vi "2 Ball Double Hot B.vi"(1 "Run?":bool) -> (0 "Done?":bool)   [LabVIEW 2013]
uses:
  Globals/Homes.vi
  Globals/Useful Values.vi
panel:
  out "Time Elapsed":dbl
  out "Sum":dbl
  out "Ready for Vision?":bool
  out "Side":dbl
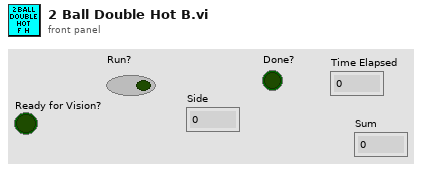
[diagram p1: front panel]
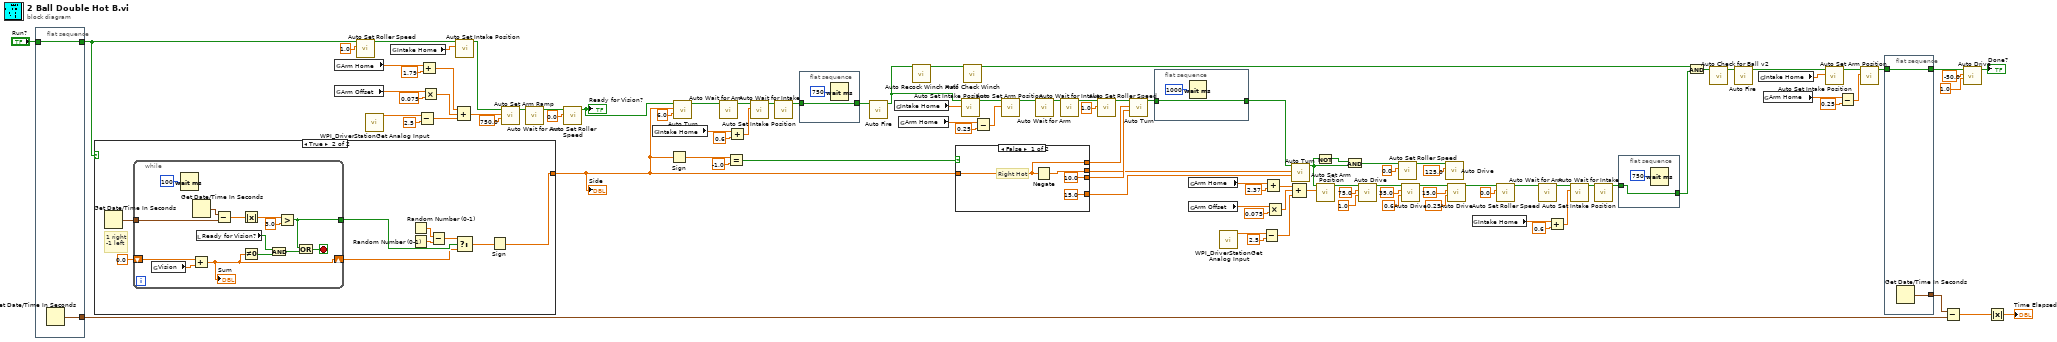
[diagram p0: block diagram]
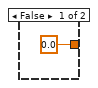
[diagram p2: hidden frame]
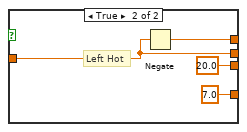
[diagram p3: hidden frame]
diagram:
  n1 = flat-sequence {
    tunnel: "Run?" -> [w107]
    tunnel: [w107] -> w49
    tunnel: [w106] -> w44
    frame #0 {
      n2 = Get Date/Time In Seconds() -> (seconds since 1Jan1904=w106:timestamp)
    }
  }
  n3 = case shown="True" w49 {
    tunnel: [0.0 w109] -> w54
    frame False {
    }
    frame True {
      # "1 right\n-1 left"
      n4 = Get Date/Time In Seconds() -> (seconds since 1Jan1904=w116:timestamp)
      n5 = while {
        shift-right: [w127] -> w111
        shift-left: 0.0 -> [w130]
        tunnel: w116 -> [w125]
        tunnel: [w118] -> w112
        stop <- w120 stop-if-true
        n6 = global read "Useful Values.vi" "Vision"() -> (w131:dbl)
        n7 = Wait (ms)(milliseconds to wait=u32 100) -> ()  [unwired: 1 out]
        n8 = Add(x=w130, y=w131) -> (x+y=w127:dbl)
        "Sum" <- w127
        n9 = Get Date/Time In Seconds() -> (seconds since 1Jan1904=w124:timestamp)
        n10 = local read "Ready for Vision?"() -> (w128:bool)
        n11 = Subtract(x=w124, y=w125) -> (x-y=w123:dbl)
        n12 = Absolute Value(x=w123) -> (abs(x)=w122:dbl)
        n13 = Not Equal To 0?(x=w127) -> (x != 0?=w126:bool)
        n14 = And(x=w128, y=w126) -> (x .and. y?=w119:bool)
        n15 = Greater?(x=w122, y=3.0) -> (0:w118:bool)
        n16 = Or(x=w118, y=w119) -> (x .or. y?=w120:bool)
      }
      n17 = Random Number (0-1)() -> (number: 0 to 1=w113:dbl)
      n18 = Random Number (0-1)() -> (number: 0 to 1=w114:dbl)
      n19 = Subtract(x=w113, y=w114) -> (x-y=w115:dbl)
      n20 = Select(t=w115, s=w112, f=w111) -> (s? t:f=w110:dbl)
      n21 = Sign(1:w110) -> (0:w109:dbl)
    }
  }
  "Side" <- w54
  n22 = global read "Homes.vi" "Arm Home"() -> (w9:dbl)
  n23 = global read "Useful Values.vi" "Arm Offset"() -> (w6:dbl)
  n24 = call "Auto Set Roller Speed.vi"("Value"=1.0, "Run?"=w49) -> ("Done"=w74:bool)  [unwired: 9 in]
  n25 = call <vilib>:"WPI_DriverStationGet Analog Input.vi"() -> ("Analog 1 (V)"=w3:dbl)  [unwired: 8 in, 3 out]
  n26 = global read "Homes.vi" "Intake Home"() -> (w104:dbl)
  n27 = Subtract(x=w3, y=2.5) -> (x-y=w2:dbl)
  n28 = Add(x=w9, y=1.79) -> (x+y=w5:dbl)
  n29 = Multiply(x=w6, y=0.075) -> (x*y=w8:dbl)
  n30 = call "Auto Set Intake Position.vi"("Intake Position"=w104, "Run?"=w74) -> ("Done"=w73:bool)  [unwired: 9 in]
  n31 = Compound Arithmetic op=ADD(w5, w8, w2) -> (w1:dbl)
  n32 = call "Auto Set Arm Ramp.vi"("Time (ms)"=750.0, "Arm Position"=w1, "Run?"=w73) -> ("Done"=w52:bool)  [unwired: 8 in]
  n33 = call "Auto Wait for Arm.vi"("Run?"=w52) -> ("Done"=w53:bool)  [unwired: 10 in]
  n34 = call "Auto Set Roller Speed.vi"("Value"=0.0, "Run?"=w53) -> ("Done"=w51:bool)  [unwired: 9 in]
  "Ready for Vision?" <- w51
  n35 = global read "Homes.vi" "Intake Home"() -> (w103:dbl)
  n36 = Sign(1:w54) -> (0:w91:dbl)
  n37 = call "Auto Turn.vi"("Turn Amount"=6.0, "+/-?"=w54, "Run?"=w51) -> ("Done"=w70:bool)  [unwired: 8 in]
  n38 = call "Auto Wait for Arm.vi"("Run?"=w70) -> ("Done"=w100:bool)  [unwired: 10 in]
  n39 = Equal?(x=w91, y=-1.0) -> (x = y?=w89:bool)
  n40 = Add(x=w103, y=0.6) -> (x+y=w102:dbl)
  n41 = call "Auto Set Intake Position.vi"("Intake Position"=w102, "Run?"=w100) -> ("Done"=w71:bool)  [unwired: 9 in]
  n42 = call "Auto Wait for Intake.vi"("Run?"=w71) -> ("Done"=w86:bool)  [unwired: 10 in]
  n43 = flat-sequence {
    tunnel: w86 -> [w132]
    tunnel: [w132] -> w77
    frame #0 {
      n44 = Wait (ms)(milliseconds to wait=u32 750) -> ()  [unwired: 1 out]
    }
  }
  n45 = call "Auto Fire.vi"("Run?"=w77) -> ("Done"=w68:bool)  [unwired: 10 in]
  n46 = global read "Homes.vi" "Intake Home"() -> (w98:dbl)
  n47 = global read "Homes.vi" "Arm Home"() -> (w81:dbl)
  n48 = call "Auto Recock Winch Half.vi"("Run?"=w68) -> ("Done"=w69:bool)  [unwired: 10 in]
  n49 = case shown="False" w89 {
    tunnel: [10.0 ("Turn Amount") 20.0 ("Turn Amount")] -> w88
    tunnel: w54 -> [w135 w138]
    tunnel: [w135 w139] -> w87
    tunnel: [w136 w138] -> w42
    tunnel: [15.0 ("Turn Amount") 7.0 ("Turn Amount")] -> w41
    frame False {
      # "Right Hot"
      n50 = Negate(x=w135) -> (-x=w136:dbl)
    }
    frame True {
      # "Left Hot"
      n51 = Negate(x=w138) -> (-x=w139:dbl)
    }
  }
  n52 = call "Auto Set Intake Position.vi"("Intake Position"=w98, "Run?"=w68) -> ("Done"=w99:bool)  [unwired: 9 in]
  n53 = call "Auto Check Winch.vi"("Run?"=w69) -> ("Done"=w33:bool)  [unwired: 10 in]
  n54 = Subtract(x=w81, y=0.25) -> (x-y=w80:dbl)
  n55 = call "Auto Set Arm Position.vi"("Arm Position"=w80, "Run?"=w99) -> ("Done"=w97:bool)  [unwired: 9 in]
  n56 = call "Auto Wait for Arm.vi"("Run?"=w97) -> ("Done"=w96:bool)  [unwired: 10 in]
  n57 = call "Auto Wait for Intake.vi"("Run?"=w96) -> ("Done"=w95:bool)  [unwired: 10 in]
  n58 = call "Auto Set Roller Speed.vi"("Value"=1.0, "Run?"=w95) -> ("Done"=w93:bool)  [unwired: 9 in]
  n59 = call "Auto Turn.vi"("Turn Amount"=w88, "+/-?"=w87, "Run?"=w93) -> ("Done"=w92:bool)  [unwired: 8 in]
  n60 = flat-sequence {
    tunnel: w92 -> [w143]
    tunnel: [w143] -> w43
    frame #0 {
      n61 = Wait (ms)(milliseconds to wait=u32 1000) -> ()  [unwired: 1 out]
    }
  }
  n62 = global read "Homes.vi" "Arm Home"() -> (w19:dbl)
  n63 = global read "Useful Values.vi" "Arm Offset"() -> (w16:dbl)
  n64 = call <vilib>:"WPI_DriverStationGet Analog Input.vi"() -> ("Analog 1 (V)"=w13:dbl)  [unwired: 8 in, 3 out]
  n65 = Subtract(x=w13, y=2.5) -> (x-y=w12:dbl)
  n66 = Add(x=w19, y=2.37) -> (x+y=w15:dbl)
  n67 = Multiply(x=w16, y=0.075) -> (x*y=w18:dbl)
  n68 = call "Auto Turn.vi"("Turn Amount"=w41, "+/-?"=w42, "Run?"=w43) -> ("Done"=w36:bool)  [unwired: 8 in]
  n69 = Compound Arithmetic op=ADD(w15, w18, w12) -> (w11:dbl)
  n70 = Not(x=w36) -> (.not. x?=w79:bool)
  n71 = call "Auto Set Arm Position.vi"("Arm Position"=w11, "Run?"=w36) -> ("Done"=w40:bool)  [unwired: 9 in]
  n72 = And(x=w79, y=w36) -> (x .and. y?=w78:bool)
  n73 = call "Auto Drive.vi"("Speed"=1.0, "Amount"=75.0, "Run?"=w40) -> ("Done"=w27:bool)  [unwired: 8 in]
  n74 = call "Auto Set Roller Speed.vi"("Value"=0.0, "Run?"=w78) -> ("Done"=w83:bool)  [unwired: 9 in]
  n75 = call "Auto Drive.vi"("Speed"=0.6, "Amount"=35.0, "Run?"=w27) -> ("Done"=w26:bool)  [unwired: 8 in]
  n76 = call "Auto Drive.vi"("Amount"=125.0, "Run?"=w83) -> ()  [unwired: 9 in, 1 out]
  n77 = call "Auto Drive.vi"("Speed"=0.25, "Amount"=15.0, "Run?"=w26) -> ("Done"=w25:bool)  [unwired: 8 in]
  n78 = global read "Homes.vi" "Intake Home"() -> (w62:dbl)
  n79 = call "Auto Set Roller Speed.vi"("Value"=0.0, "Run?"=w25) -> ("Done"=w38:bool)  [unwired: 9 in]
  n80 = call "Auto Wait for Arm.vi"("Run?"=w38) -> ("Done"=w55:bool)  [unwired: 10 in]
  n81 = Add(x=w62, y=0.6) -> (x+y=w66:dbl)
  n82 = call "Auto Set Intake Position.vi"("Intake Position"=w66, "Run?"=w55) -> ("Done"=w56:bool)  [unwired: 9 in]
  n83 = call "Auto Wait for Intake.vi"("Run?"=w56) -> ("Done"=w57:bool)  [unwired: 10 in]
  n84 = flat-sequence {
    tunnel: w57 -> [w144]
    tunnel: [w144] -> w34
    frame #0 {
      n85 = Wait (ms)(milliseconds to wait=u32 750) -> ()  [unwired: 1 out]
    }
  }
  n86 = And(x=w33, y=w34) -> (x .and. y?=w32:bool)
  n87 = call "Auto Check for Ball v2.vi"("Run?"=w32) -> ("Done"=w35:bool)  [unwired: 10 in]
  n88 = call "Auto Fire.vi"("Run?"=w35) -> ("Done"=w65:bool)  [unwired: 10 in]
  n89 = global read "Homes.vi" "Intake Home"() -> (w61:dbl)
  n90 = global read "Homes.vi" "Arm Home"() -> (w59:dbl)
  n91 = call "Auto Set Intake Position.vi"("Intake Position"=w61, "Run?"=w65) -> ("Done"=w64:bool)  [unwired: 9 in]
  n92 = Subtract(x=w59, y=0.25) -> (x-y=w60:dbl)
  n93 = call "Auto Set Arm Position.vi"("Arm Position"=w60, "Run?"=w64) -> ("Done"=w48:bool)  [unwired: 9 in]
  n94 = flat-sequence {
    tunnel: w48 -> [w147]
    tunnel: [w147] -> w24
    tunnel: [w146] -> w47
    frame #0 {
      n95 = Get Date/Time In Seconds() -> (seconds since 1Jan1904=w146:timestamp)
    }
  }
  n96 = Subtract(x=w47, y=w44) -> (x-y=w46:dbl)
  n97 = call "Auto Drive.vi"("Speed"=1.0, "Amount"=-50.0, "Run?"=w24) -> ("Done"=→"Done?":bool)  [unwired: 8 in]
  n98 = Absolute Value(x=w46) -> (abs(x)=→"Time Elapsed":dbl)
